vi "svx_Orbit CheckboxToIndex.vi"(4 "All Children Tags":string[](array[string]), 6 "All parents Tags":string[](array[string]), 10 "Coords":T1, 11 "Tree ref in":refnum<vi>) -> (0 "State Changed?":bool, 2 "index":cluster{"RowIdx":i32, "ColumnIdx":i32}[](array[cluster]), 3 "Tree ref out":refnum<vi>)   [LabVIEW 2017, in "SVX Orbit.xctl"]
uses:
  <vilib>/addons/_XControls/Orbit Plot/SVX Orbit.xctl
  <vilib>/Utility/miscctls.llb/LVPoint32TypeDef.ctl
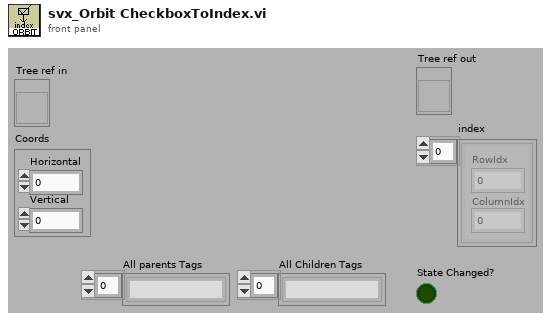
[diagram p1: front panel]
types:
  T1 = typedef "LVPoint32TypeDef.ctl" = cluster{"Horizontal":i32, "Vertical":i32}
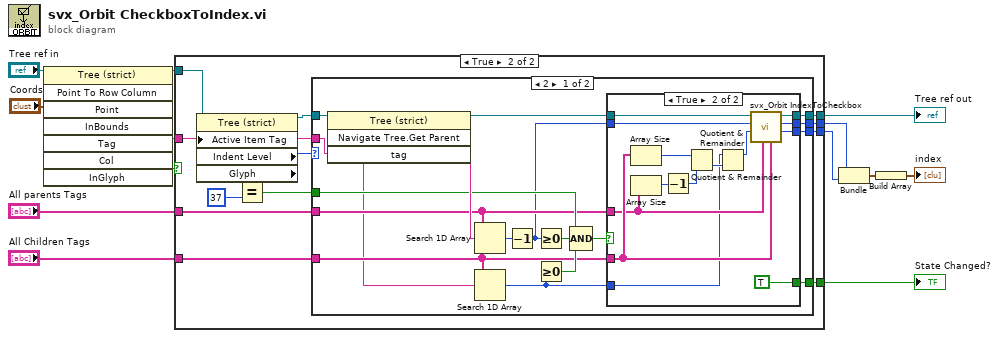
[diagram p0: block diagram]
diagram:
  n1 = invoke on="Invoke Node" class="Tree (strict)" method="Point To Row Column"(reference="Tree ref in", "Point"="Coords") -> (reference out=w13:refnum<vi>, "Tag"=w12:string, "InGlyph"=w11:bool)  [unwired: 6 in, 5 out]
  n2 = case shown="True" w11 {
    tunnel: w13 -> [w14 w27]
    tunnel: w12 -> [_ w25]
    tunnel: "All parents Tags" -> [_ w21]
    tunnel: "All Children Tags" -> [_ w20]
    tunnel: [_ w18] -> w4
    tunnel: [_ w17] -> w3
    tunnel: [w14 w16] -> w7
    tunnel: [_ w15] -> w6
    frame False {
    }
    frame True {
      n3 = property class="Tree (strict)"(reference=w27, "Active Item Tag"=w25) -> (reference out=w26:refnum<vi>, "Indent Level"=w23:i32, "Glyph"=w22:i32)  [unwired: 1 in, 1 out]
      n4 = Equal?(x=w22, y=37) -> (x = y?=w19:bool)
      n5 = case shown="2" w23 {
        tunnel: w26 -> [w44 w58]
        tunnel: w25 -> [w29 _]
        tunnel: w21 -> [w37 _]
        tunnel: w20 -> [w36 _]
        tunnel: w19 -> [w38 _]
        tunnel: [w33 _] -> w18
        tunnel: [w32 _] -> w17
        tunnel: [w31 w58] -> w16
        tunnel: [w30 _] -> w15
        frame 2 {
          n6 = invoke on="Invoke Node" class="Tree (strict)" method="Navigate Tree.Get Parent"(reference=w44, "tag"=w29) -> (reference out=w39:refnum<vi>, "Navigate Tree:Get Parent"=w43:string)  [unwired: 2 in, 2 out]
          n7 = Search 1D Array(1D array=w37, element=w43) -> (index of element=w42:i32)  [unwired: 1 in]
          n8 = Search 1D Array(1D array=w36, element=w29) -> (index of element=w28:i32)  [unwired: 1 in]
          n9 = Decrement(x=w42) -> (x-1=w34:i32)
          n10 = Greater Or Equal To 0?(x=w34) -> (x >= 0?=w41:bool)
          n11 = Greater Or Equal To 0?(x=w28) -> (x >= 0?=w40:bool)
          n12 = Compound Arithmetic op=AND(w38, w41, w40) -> (w35:bool)
          n13 = case shown="True" w35 {
            tunnel: w39 -> [w45 w57]
            tunnel: w37 -> [_ w50]
            tunnel: w36 -> [_ w56]
            tunnel: w34 -> [_ w54]
            tunnel: [_ w54] -> w33
            tunnel: [_ w53] -> w32
            tunnel: [w45 w52] -> w31
            tunnel: [_ TRUE ("State Changed?")] -> w30
            tunnel: w28 -> [_ w46]
            frame False {
            }
            frame True {
              n14 = Array Size(array=w56) -> (size(s)=w47:i32)
              n15 = Array Size(array=w50) -> (size(s)=w49:i32)
              n16 = Decrement(x=w49) -> (x-1=w48:i32)
              n17 = Quotient & Remainder(x=w47, y=w48) -> (floor(x/y)=w55:i32)  [unwired: 1 out]
              n18 = Quotient & Remainder(x=w46, y=w55) -> (x-y*floor(x/y)=w53:i32)  [unwired: 1 out]
              n19 = call <vilib>:"svx_Orbit IndexToCheckbox.vi"("All Children Tags"=w56, "All parents Tags"=w50, "ColumnIdx"=w53, "RowIdx"=w54, "Tree ref in"=w57) -> ("Tree ref out"=w52:refnum<vi>)  [unwired: 6 in]
            }
          }
        }
        frame Default {
        }
      }
    }
  }
  "Tree ref out" <- w7
  "State Changed?" <- w6
  n20 = Bundle(w4, w3) -> (w2:cluster{i32, i32})  [unwired: 1 in]
  n21 = Build Array(w2) -> (→"index":cluster{i32, i32}[])
